vi "AuMT8852B Transmitter Power.vi"(5 "Power (-40 dBm)":dbl=-40.0 format="%.2f", 7 "Set/Get (Set)":enum16{"Set", "Get"}(ring), 8 "error in (no error)":errorcluster, 10 "Script (3)":i32=3, 11 "VISA session":refnum<visa-resource-name>) -> (0 "error out":errorcluster, 2 "error code":i32, 3 "VISA session out":refnum<visa-resource-name>, 4 "Power out":dbl=-40.0 format="%.2f")   [LabVIEW 2017]
doc: "Anritsu MT8852B Bluetooth Tester\n\nSets the power level (-80 to 0 dBm) to be used for the current script. This setting takes immediate effect, even if a test is running.\n\nINPUTS\nSet/Get - whether the value is being sent to or retrieved from the instrument.\nScript - script number for which this command applies.\nPower - TX power to be used for this script.\n\nOUTPUTS\nPower out - the current TX power being used for this script."
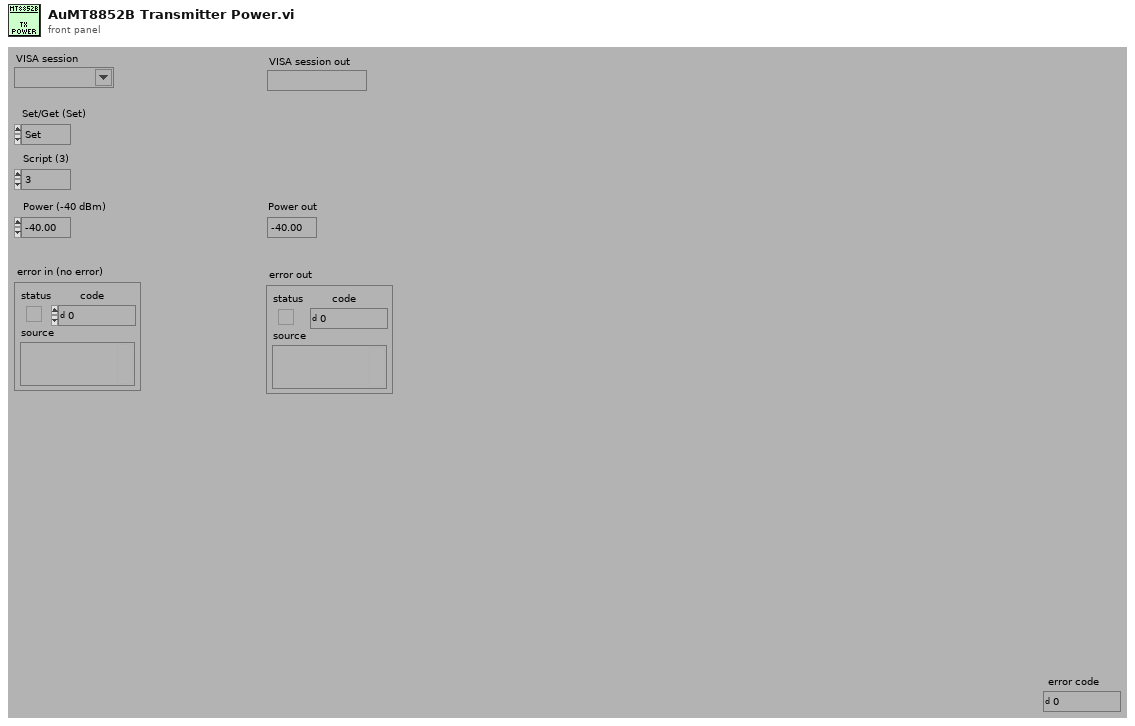
[diagram p1: front panel]
types:
  T1 = enum16{"Simulate", "Range check", "Cache", "Query instrument status"}
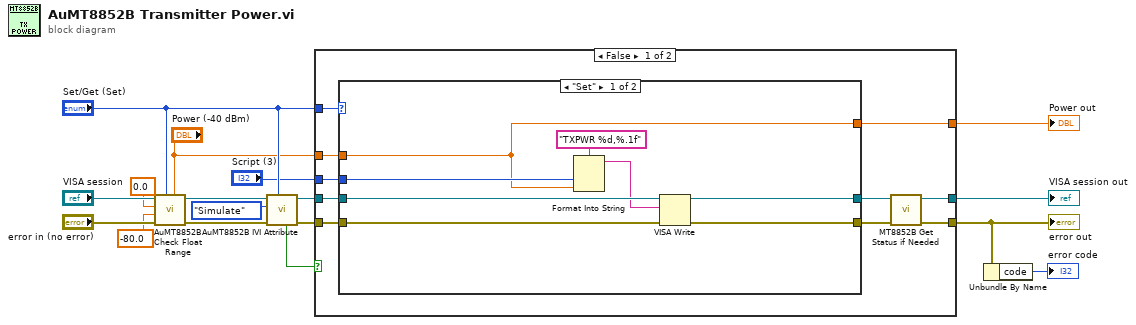
[diagram p0: block diagram]
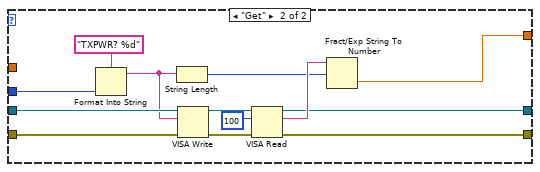
[diagram p2: hidden frame]
diagram:
  n1 = call <instrlib>:"AuMT8852B Check Float Range.vi"("Value (0)"="Power (-40 dBm)", "Set/Get (Set)"="Set/Get (Set)", "error in (no error)"="error in (no error)", "Lower limit (-1)"=-80.0, "Upper limit (1)"=0.0, "VISA session"="VISA session") -> ("error out"=w10:errorcluster, "VISA session out"=w11:refnum<visa-resource-name>)  [unwired: 4 in]
  n2 = call <instrlib>:"AuMT8852B IVI Attribute.vi"("Set/Get (Set)"="Set/Get (Set)", "error in (no error)"=w10, "Flag (Simulate)"=T1."Simulate", "VISA session"=w11) -> ("error out"=w15:errorcluster, "VISA session out"=w16:refnum<visa-resource-name>, "Value out"=w3:bool)  [unwired: 5 in]
  n3 = case shown="False" w3 {
    tunnel: "Set/Get (Set)" -> [w27 _]
    tunnel: [w20 w50] -> w5
    tunnel: [w21 w51] -> w17
    tunnel: w16 -> [w26 w51]
    tunnel: w15 -> [w25 w50]
    tunnel: [w24 w49] -> w14
    tunnel: "Script (3)" -> [w19 _]
    tunnel: "Power (-40 dBm)" -> [w18 w49]
    frame False {
      n4 = case shown="\"Set\"" w27 {
        tunnel: [w32 w36] -> w22
        tunnel: [w33 w37] -> w23
        tunnel: w26 -> [w35 w48]
        tunnel: w25 -> [w34 w47]
        tunnel: [w28 w42] -> w24
        tunnel: w19 -> [w29 w39]
        tunnel: w18 -> [w28 _]
        frame "Set" {
          n5 = Format Into String(format string="TXPWR %d,%.1f" ("Format String"), w29, w28) -> (resulting string=w30:string)  [unwired: 2 in, 1 out]
          n6 = VISA Write(VISA resource name=w35, write buffer=w30, error in (no error)=w34) -> (VISA resource name out=w33:refnum<visa-resource-name>, error out=w32:errorcluster)  [unwired: 1 out]
        }
        frame "Get" {
          n7 = Format Into String(format string="TXPWR? %d" ("Format String"), w39) -> (resulting string=w38:string)  [unwired: 2 in, 1 out]
          n8 = String Length(string=w38) -> (length=w41:i32)
          n9 = VISA Write(VISA resource name=w48, write buffer=w38, error in (no error)=w47) -> (VISA resource name out=w46:refnum<visa-resource-name>, error out=w44:errorcluster)  [unwired: 1 out]
          n10 = VISA Read(VISA resource name=w46, byte count=u32 100 ("byte count (0)"), error in (no error)=w44) -> (VISA resource name out=w37:refnum<visa-resource-name>, read buffer=w43:string, error out=w36:errorcluster)  [unwired: 1 out]
          n11 = Fract/Exp String To Number(string=w43, offset=w41) -> (number=w42:dbl)  [unwired: 2 in, 1 out]
        }
      }
      n12 = call <instrlib>:"MT8852B Get Status if Needed.vi"("error in (no error)"=w22, "VISA session"=w23) -> ("error out"=w20:errorcluster, "VISA session out"=w21:refnum<visa-resource-name>)  [unwired: 8 in]
    }
    frame True {
    }
  }
  "error out" <- w5
  "VISA session out" <- w17
  "Power out" <- w14
  n13 = Unbundle By Name(w5) -> ("code"=→"error code":i32)
